vi "Send Request To Execution Engine.vi"(0 "Request Message":string, 5 "Request Header":string, 9 "Request Content Type":i32(ring) items=["Info", "Warning", "Error", "Action"], 11 "error in (no error)":errorcluster) -> (4 "Response":string, 15 "error out":errorcluster)   [LabVIEW 2023, in "RFCalAndFixtureCharact.Common.lvlib"]
uses:
  RFCalAndFixtureCharact.Common.lvlib
  C:/srd-semi-rfcal-software/AuxTools/STSRFFixtureCharactUtility/Source/Code Modules/Dependencies/NationalInstruments.RFCalibration.ExecutionEngine.dll
  Dependencies/NationalInstruments.RFCalibration.ExecutionEngine.dll
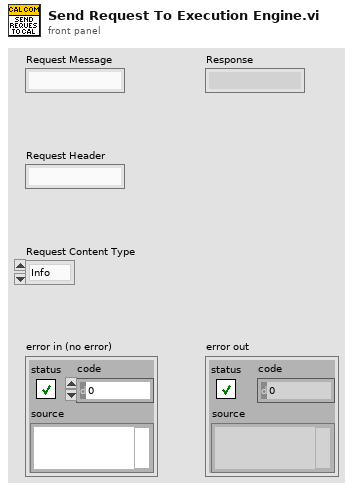
[diagram p1: front panel]
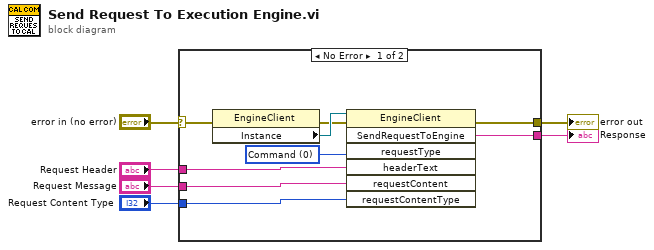
[diagram p0: block diagram]
diagram:
  n1 = case shown="No Error" "error in (no error)" {
    selector: "error in (no error)" -> [w11 w16]
    tunnel: [w15 w16] -> w6
    tunnel: [w14 _] -> w5
    tunnel: "Request Header" -> [w10 _]
    tunnel: "Request Message" -> [w9 _]
    tunnel: "Request Content Type" -> [w7 _]
    frame No Error {
      w8 = 0 items=["Command", "ResultConfirmation", "CheckListenerStatus", "IntermediateResultReview"] ("requestType")
      n2 = property class="EngineClient"(error in=w11) -> (error out=w12:errorcluster, "Instance"=w13:refnum<k24>)  [unwired: 1 in, 1 out]
      n3 = invoke class="EngineClient" method="SendRequestToEngine"(reference=w13, error in=w12, "requestType"=w8, "headerText"=w10, "requestContent"=w9, "requestContentType"=w7) -> (error out=w15:errorcluster, "SendRequestToEngine"=w14:string)  [unwired: 1 in, 5 out]
    }
    frame Error {
    }
  }
  "error out" <- w6
  "Response" <- w5
